vi "SetTile.vi"(8 "error in (no error)":errorcluster, 9 "Coordinates":T1, 10 "TileNumber":u32, 11 "Game in":refnum<class "Game.lvclass">) -> (0 "error out":errorcluster, 3 "Game out":refnum<class "Game.lvclass">)   [LabVIEW 2019, in "RT_Game.lvlib" / "Game.lvclass"]
uses:
  Game.lvclass
  Coordinate.ctl
  Engine/SetTileData.ctl
  Engine/MessageCluster.ctl
  Game.lvclass/Game.ctl
  Engine/Engine.lvclass
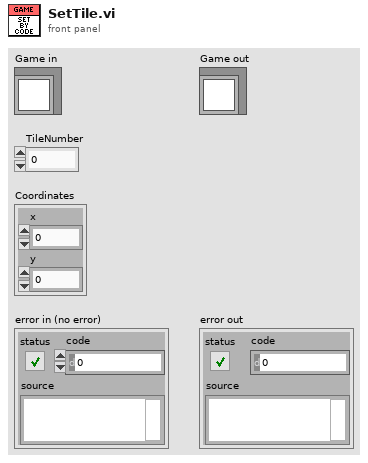
[diagram p1: front panel]
types:
  T1 = typedef "RT_Game.lvlib/Game.lvclass/Coordinate.ctl" = cluster{"x":dbl, "y":dbl}
  T2 = typedef "RT_Game.lvlib/Engine.lvclass/MessageCluster.ctl" = cluster{"Message":string, "Data":variant}
  T3 = typedef "RT_Game.lvlib/Engine.lvclass/SetTileData.ctl" = cluster{"TileCode":u32, "Position":T1}
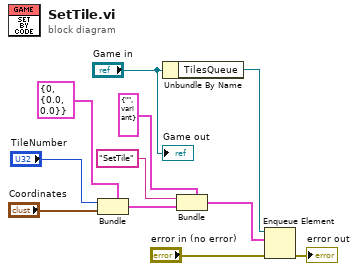
[diagram p0: block diagram]
diagram:
  n1 = Bundle(cluster=T3 {"TileCode"=0, "Position"={"x"=0.0, "y"=0.0}} ("SetTileData"), "TileCode"="TileNumber", "Position"="Coordinates") -> (w1:T3)
  n2 = Unbundle By Name("Game in") -> ("TilesQueue"=w6:refnum<queue>)
  n3 = Bundle(cluster=T2 {"Message"="", "Data"=variant} ("element"), "Message"="SetTile", "Data"=w1) -> (w4:T2)
  n4 = Enqueue Element(queue=w6, element=w4, error in (no error)="error in (no error)") -> (error out=→"error out":errorcluster)  [unwired: 1 in, 2 out]
  "Game out" <- "Game in"
